vi "testXctrl.vi"() -> ()   [LabVIEW 2014]
uses:
  Robot2015.xctl
panel:
  in  "NBTotesUnder":u8
  out "Robot2015":dbl(xcontrol)
  in  "Offset":enum16{"Step", "platform", "Ground"}(ring)
  in  "Container?":bool
  in  "position":dbl
  in  "stop":bool
  in  "Opening":enum16{"Close", "Narrow", "Wide"}(ring)
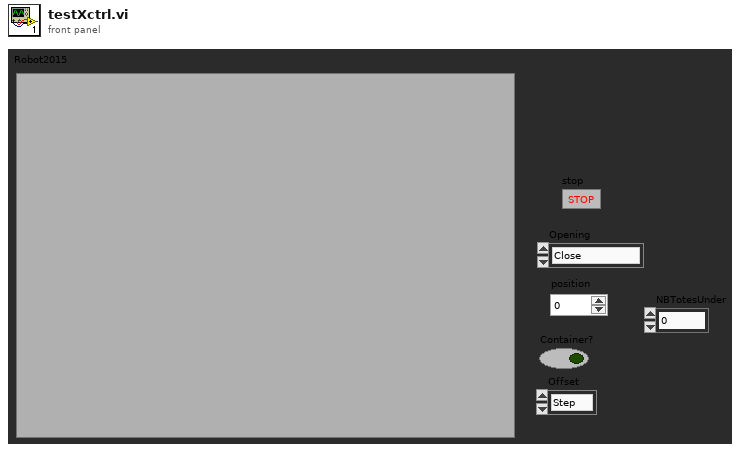
[diagram p1: front panel]
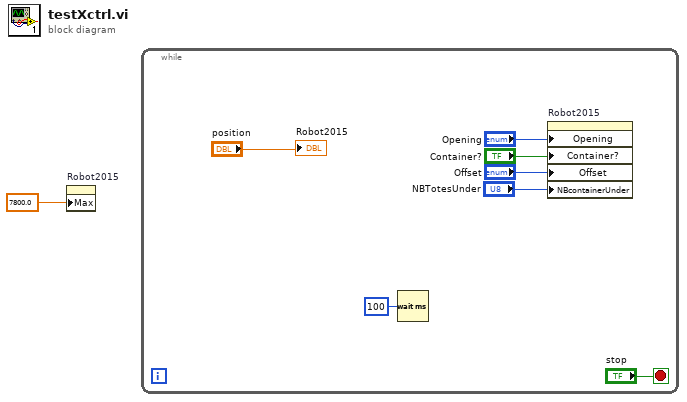
[diagram p0: block diagram]
diagram:
  n1 = property on="Robot2015" class="Robot2015 (strict)"("Max"=7800.0) -> ()  [unwired: 2 in, 2 out]
  n2 = while {
    stop <- "stop" stop-if-true
    n3 = Wait (ms)(milliseconds to wait=u32 100) -> ()  [unwired: 1 out]
    n4 = property on="Robot2015" class="Robot2015 (strict)"("Opening"="Opening", "Container?"="Container?", "Offset"="Offset", "NBcontainerUnder"="NBTotesUnder") -> ()  [unwired: 2 in, 2 out]
    "Robot2015" <- "position"
  }
